vi "User-Defined Test Basic.vi"() -> (3 "Unit Test Framework Results":T1)   [LabVIEW 2025]
doc: "Demonstrates how to use the User-defined Test Template.vit file to create a basic user-defined test VI. This test VI returns only the test results."
uses:
  <vilib>/utf/common/utf_test_result_troll.ctl
  <vilib>/utf/common/utf_test_result.ctl
  <vilib>/utf/common/utf_test_result_failure.ctl
  <vilib>/utf/common/utf_test_comparison_operators.ctl
  <vilib>/utf/common/utf_vi_tag.ctl
  <vilib>/utf/NI_UnitTestFramework.lvlib
panel:
  # "Overview: Demonstrates how to use the User-defined Test Template.vit file to create a basic user-defined test VI. This test VI returns only the test results."
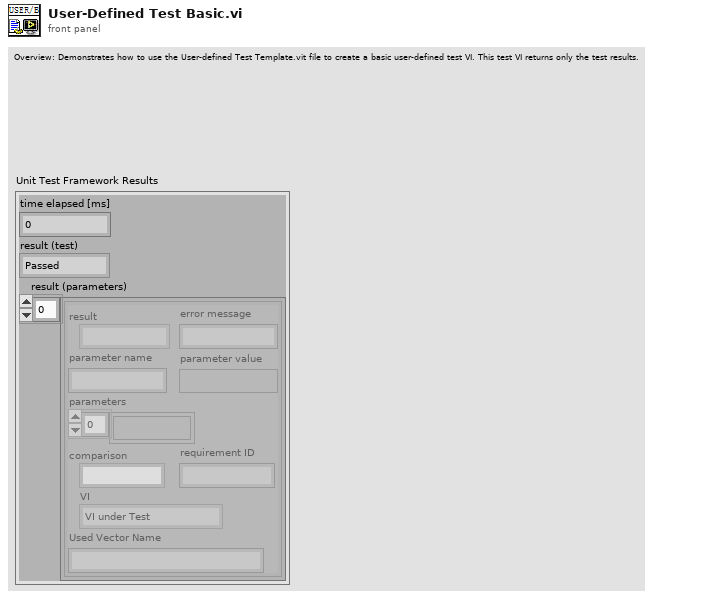
[diagram p1: front panel]
types:
  T1 = typedef "NI_UnitTestFramework.lvlib/utf_test_result_troll.ctl" = cluster{"time elapsed [ms]":u32, "result (test)":T2, "result (parameters)":T3[]}
  T2 = typedef "NI_UnitTestFramework.lvlib/utf_test_result.ctl" = enum16{"Passed", "Failed", "Error", "Skipped", "Not Processed"}
  T3 = typedef "NI_UnitTestFramework.lvlib/utf_test_result_failure.ctl" = cluster{"result":T2, "error message":string, "parameter name":string, "parameter value":variant, "parameters":variant[], "comparison":T4, "requirement ID":string, "VI":T5, "Used Vector Name":string}
  T4 = typedef "NI_UnitTestFramework.lvlib/utf_test_comparison_operators.ctl" = enum16{"=", "!=", ">", ">=", "<", "<=", "range", "symmetric tolerance", "asymmetric tolerance", "string contains", "string not contain", "array size", "string length", "array range", "by element", "array range (limit array)", "user-defined", "array contains", "array not contain", "vector length", "= (elm)", "!= (elm)", "= (case insensitive)", "!= (case insensitive)"}
  T5 = typedef "NI_UnitTestFramework.lvlib/utf_vi_tag.ctl" = enum16{"Setup VI", "VI under Test", "Teardown VI"}
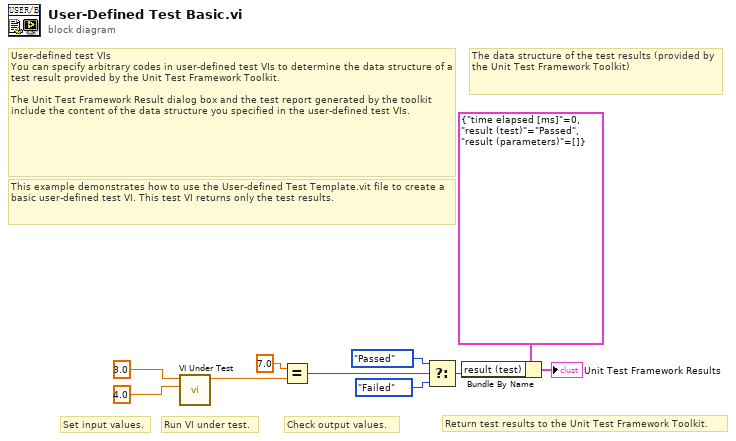
[diagram p0: block diagram]
diagram:
  # "User-defined test VIs\nYou can specify arbitrary codes in user-defined test VIs to determine the data structure of a test result provided by the Unit Test Framework Toolkit.\n\nThe Unit Test Framework Result dialog box and the test report generated by the toolkit include the content of the data structure you specified in the user-defined test VIs."
  # "The data structure of the test results (provided by the Unit Test Framework Toolkit)"
  # "This example demonstrates how to use the User-defined Test Template.vit file to create a basic user-defined test VI. This test VI returns only the test results."
  # "Return test results to the Unit Test Framework Toolkit."
  # "Check output values."
  # "Run VI under test."
  # "Set input values."
  n1 = call "VI Under Test.vi"("N2"=4.0 ("Y"), "N1"=3.0 ("X")) -> ("Result"=w1:dbl)  [unwired: 1 in, 8 out]
  n2 = Equal?(x=7.0 ("X"), y=w1) -> (x = y?=w8:bool)
  n3 = Select(t=utf_test_result."Passed" ("Result (Test)"), s=w8, f=utf_test_result."Failed" ("Result (Test)")) -> (s? t:f=w5:T2)
  n4 = Bundle By Name(cluster=T1 {"time elapsed [ms]"=0, "result (test)"=enum."Passed", "result (parameters)"=[]} ("Constant"), "result (test)"=w5) -> (→"Unit Test Framework Results":T1)
